vi "Read Funds Dispensed.vi"(8 "error in (no error)":errorcluster, 11 "Simulated Sensor Interface Actor in":refnum<class "Simulated Sensor Interface Actor.lvclass">) -> (0 "error out":errorcluster, 3 "Simulated Sensor Interface Actor out":refnum<class "Simulated Sensor Interface Actor.lvclass">)   [LabVIEW 2019]
uses:
  <vilib>/ActorFramework/Actor/Actor.lvclass
  Simulated Sensor Interface Actor.lvclass
  C:/Workspace/CLA/ATM AF/Sensor Interface Actor/Sensor Interface Actor/Sensor Interface Actor.lvclass
  C:/Program Files (x86)/National Instruments/LabVIEW 2019/vi.lib/ActorFramework/Actor/Actor.lvclass
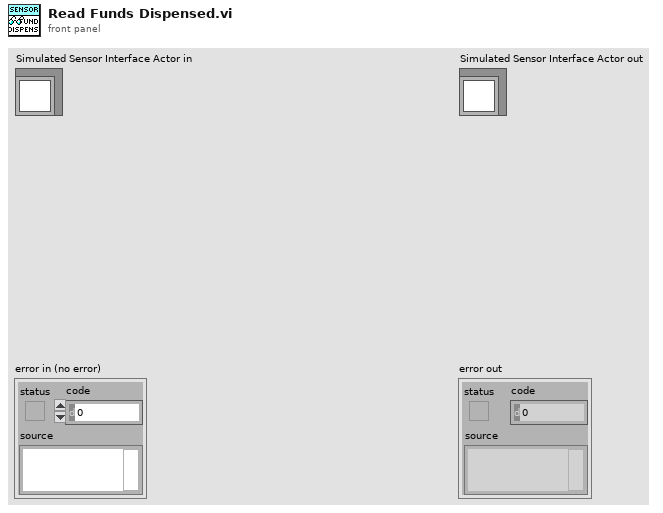
[diagram p1: front panel]
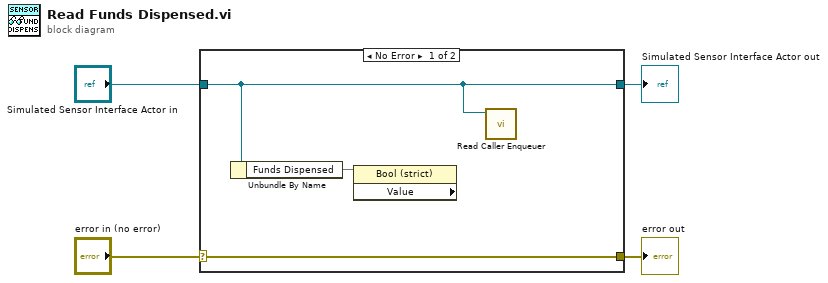
[diagram p0: block diagram]
diagram:
  n1 = case shown="No Error" "error in (no error)" {
    selector: "error in (no error)" -> [w7 w8]
    tunnel: [w7 w8] -> w3
    tunnel: [w5 w9] -> w1
    tunnel: "Simulated Sensor Interface Actor in" -> [w5 w9]
    frame No Error {
      n2 = Unbundle By Name(w5) -> ("Funds Dispensed"=w6)
      n3 = property class="Bool (strict)" props=["Value"](reference=w6) -> ()  [unwired: 1 in, 3 out]
      n4 = call <vilib>:"Read Caller Enqueuer.vi"("Actor"=w5) -> ()  [unwired: 10 in, 1 out]
    }
    frame Error {
    }
  }
  "error out" <- w3
  "Simulated Sensor Interface Actor out" <- w1
